vi "HighlightPoint.vi"(2 "error in":errorcluster, 3 "Image In":T1, 4 "index":i32, 5 "points":cluster{"Edge Info":T2, "Boolean":bool}[](array[cluster]) {"Edge Info"."Distance (Real-World)" format="%.2f"; "Edge Info"."Location (Real-World)"."Y" format="%.2g"; "Edge Info"."Location (Real-World)"."X" format="%.2f"; "Edge Info"."Noise" format="%.2f"; "Edge Info"."Location (Pixel)"."Y" format="%.2g"; "Edge Info"."Location (Pixel)"."X" format="%.2f"; "Edge Info"."Strength" format="%.2f"; "Edge Info"."Distance (Pixel)" format="%.2f"}) -> (0 "error out":errorcluster, 1 "Image Out":T1)   [LabVIEW 2014]
uses:
  <vilib>/vision/Measure.llb/Edge New.ctl
  <vilib>/vision/Image Controls.llb/IMAQ Image.ctl
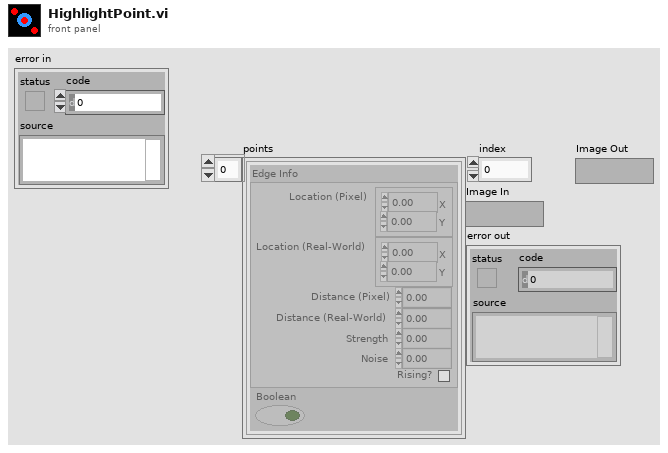
[diagram p1: front panel]
types:
  T1 = typedef "IMAQ Image.ctl" = refnum<image>
  T2 = typedef "Edge New.ctl" = cluster{"Location (Pixel)":cluster{"X":sgl, "Y":sgl}, "Location (Real-World)":cluster{"X":sgl, "Y":sgl}, "Distance (Pixel)":dbl, "Distance (Real-World)":dbl, "Strength":dbl, "Noise":dbl, "Rising?":bool}
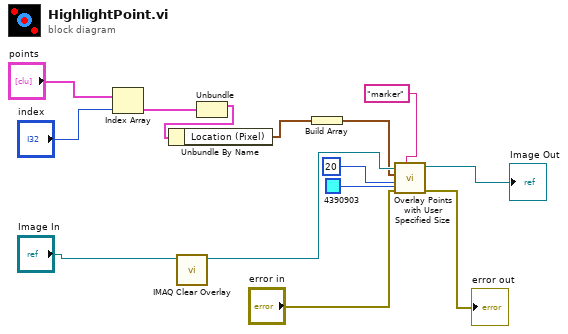
[diagram p0: block diagram]
diagram:
  n1 = Index Array(array="points", index="index") -> (element=w14:cluster{"Edge Info":T2, "Boolean":bool})
  n2 = call "IMAQ Clear Overlay"("Image"="Image In") -> ("Image Out"=w9:T1)  [unwired: 9 in, 1 out]
  n3 = Unbundle(w14) -> ("Edge Info"=w13:T2)  [unwired: 1 out]
  n4 = Unbundle By Name(w13) -> ("Location (Pixel)"=w4:cluster{"X":sgl, "Y":sgl})
  n5 = Build Array(w4) -> (w3:cluster{"X":sgl, "Y":sgl}[])
  n6 = call "Overlay Points with User Specified Size.vi"("Color"=u32 4390903, "Group"="marker", "error in"="error in", "Point Diameter (5)"=u32 20, "Points"=w3, "Image In"=w9) -> ("error out"=→"error out":errorcluster, "Image Out"=→"Image Out":T1)  [unwired: 4 in]
